vi "CPLX_EXT.vi"(4 "Value":cxt) -> (1 "Constant":refnum<class "Abs_Complex Extended Float.lvclass">)   [LabVIEW 2021, in "Const_CPLX_EXT.lvclass"]
uses:
  Const_CPLX_EXT.lvclass
  Abs_Types/Complex Extended Float/Abs_Complex Extended Float.lvclass
  C:/Program Files (x86)/National Instruments/LabVIEW 2021/vi.lib/TSA/Abstract Data Classes/Abs_Types/Complex Extended Float/Abs_Complex Extended Float.lvclass
  Const_CPLX_EXT.lvclass/Const_CPLX_EXT.ctl
  Properties/Write Value.vi
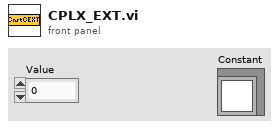
[diagram p1: front panel]
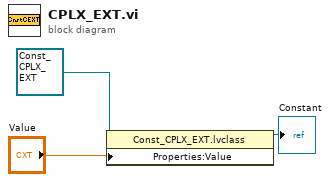
[diagram p0: block diagram]
diagram:
  n1 = property class="Const_CPLX_EXT.lvclass"(reference=refnum<class "Const_CPLX_EXT.lvclass"> refnum ("Constants.lvlib:Numeric.lvclass"), "Properties:Value"="Value") -> (reference out=→"Constant":refnum<class "Const_CPLX_EXT.lvclass">)  [unwired: 1 in, 1 out]
